vi "Initiate Sampling.vi"(7 "display string (none)":string, 8 "error in":errorcluster, 9 "stream mode (False)":bool, 10 "ARM mode (SGL)":T1=enum."SGL", 11 "VISA resource in":refnum<visa-resource-name>) -> (0 "error out":errorcluster, 3 "VISA resource out":refnum<visa-resource-name>)   [LabVIEW 2018, in "3458A Virtual Digitizer.lvlib" / "3458A Digitizing Low Levels.lvlib"]
doc: "Arms DMM so it may start digitizing depending on the mode setting. \n\nNote: Reentrant VI so it can be executed in parallel for multiple 3458A sessions."
uses:
  3458A Digitizing Low Levels.lvlib
  Configure/First Sample Trigger.ctl
  3458A Basic Driver/3458A Basic Driver.lvlib
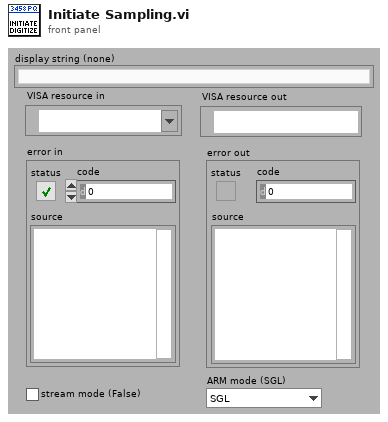
[diagram p1: front panel]
types:
  T1 = typedef "3458A Virtual Digitizer.lvlib/3458A Digitizing Low Levels.lvlib/First Sample Trigger.ctl" = enum16{"AUTO", "EXT", "SYN", "SGL", "HOLD", "LEVEL"}
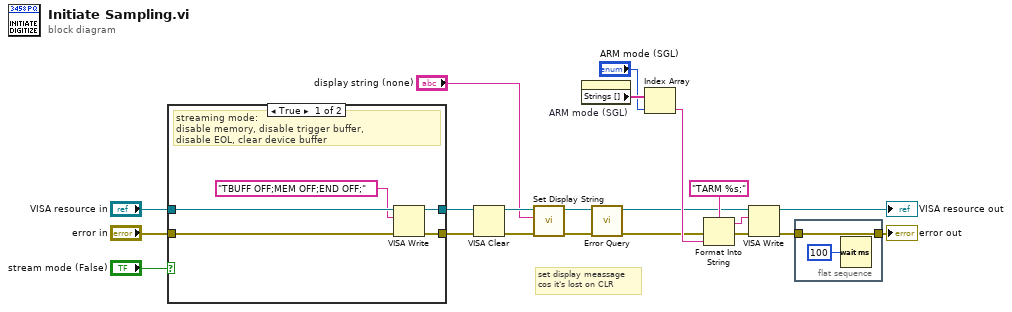
[diagram p0: block diagram]
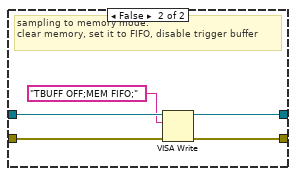
[diagram p2: hidden frame]
diagram:
  # "set display meassage\ncos it's lost on CLR"
  n1 = case shown="True" "stream mode (False)" {
    tunnel: "error in" -> [w26 w31]
    tunnel: "VISA resource in" -> [w25 w30]
    tunnel: [w22 w27] -> w10
    tunnel: [w23 w28] -> w11
    frame True {
      # "streaming mode:\ndisable memory, disable trigger buffer,\ndisable EOL, clear device buffer"
      n2 = VISA Write(VISA resource name=w25, write buffer="TBUFF OFF;MEM OFF;END OFF;", error in (no error)=w26) -> (VISA resource name out=w22:refnum<visa-resource-name>, error out=w23:errorcluster)  [unwired: 1 out]
    }
    frame False {
      # "sampling to memory mode:\nclear memory, set it to FIFO, disable trigger buffer"
      n3 = VISA Write(VISA resource name=w30, write buffer="TBUFF OFF;MEM FIFO;", error in (no error)=w31) -> (VISA resource name out=w27:refnum<visa-resource-name>, error out=w28:errorcluster)  [unwired: 1 out]
    }
  }
  n4 = VISA Clear(VISA resource name=w10, error in (no error)=w11) -> (VISA resource name out=w8:refnum<visa-resource-name>, error out=w9:errorcluster)
  n5 = call "Set Display String.vi"("error in(no error)"=w9, "display string (none)"="display string (none)", "VISA Resource Name"=w8) -> ("error out"=w6:errorcluster, "VISA resource name out"=w5:refnum<visa-resource-name>)  [unwired: 7 in]
  n6 = property on="ARM mode (SGL)" class="Enum (strict)"() -> ("Strings []"=w18:string[])  [unwired: 2 in, 2 out]
  n7 = call "Error Query.vi"("error in (no error)"=w6, "VISA resource name"=w5) -> ("error out"=w3:errorcluster, "VISA resource name out"=w4:refnum<visa-resource-name>)  [unwired: 6 in, 2 out]
  n8 = Index Array(array=w18, index="ARM mode (SGL)") -> (element=w13:string)
  n9 = Format Into String(format string="TARM %s;" ("write buffer"), error in=w3, w13) -> (resulting string=w14:string, error out=w16:errorcluster)  [unwired: 1 in]
  n10 = VISA Write(VISA resource name=w4, write buffer=w14, error in (no error)=w16) -> (VISA resource name out=→"VISA resource out":refnum<visa-resource-name>, error out=w2:errorcluster)  [unwired: 1 out]
  n11 = flat-sequence {
    tunnel: [w33] -> w1
    tunnel: w2 -> [w33]
    frame #0 {
      n12 = Wait (ms)(milliseconds to wait=u32 100) -> ()  [unwired: 1 out]
    }
  }
  "error out" <- w1
